vi "MQTT_PubAck_Read.vi"(8 "error in (no error)":errorcluster, 11 "SSL_Connection":T1) -> (0 "error out":errorcluster, 2 "Message ID":u16=10 format="%x", 3 "SSL_Connection":T1)   [LabVIEW 2018, in "AWS_IoT.lvlib"]
doc: "© 2015 - daq.io, LLC - Peter Adelhardt"
uses:
  AWS_IoT.lvlib
  Controls/SSL_Connection.ctl
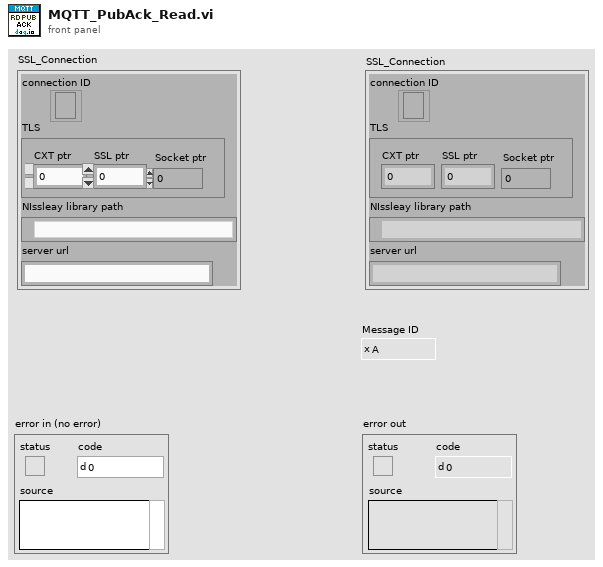
[diagram p1: front panel]
types:
  T1 = typedef "AWS_IoT.lvlib/SSL_Connection.ctl" = cluster{"connection ID":refnum<k5>, "TLS":cluster{"CXT ptr":i32, "SSL ptr":i32, "Socket ptr":i32}, "NIssleay library path":path, "server url":string}
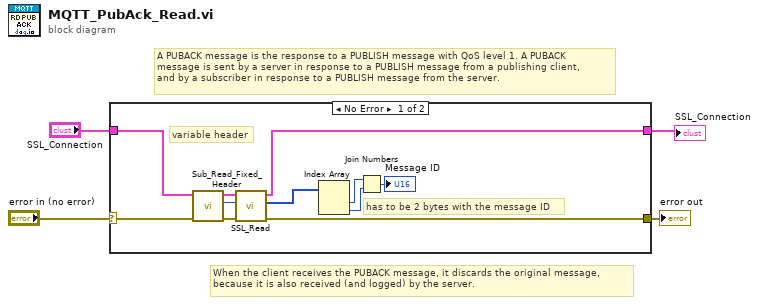
[diagram p0: block diagram]
diagram:
  # "When the client receives the PUBACK message, it discards the original message,\nbecause it is also received (and logged) by the server."
  # "A PUBACK message is the response to a PUBLISH message with QoS level 1. A PUBACK\nmessage is sent by a server in response to a PUBLISH message from a publishing client,\nand by a subscriber in response to a PUBLISH message from the server."
  n1 = case shown="No Error" "error in (no error)" {
    selector: "error in (no error)" -> [w15 w17]
    tunnel: [w8 w17] -> w3
    tunnel: "SSL_Connection" -> [w6 w16]
    tunnel: [w5 w16] -> w1
    frame No Error {
      # "has to be 2 bytes with the message ID"
      # "variable header"
      n2 = call "Sub_Read_Fixed_Header.vi"("error in (no error)"=w15, "SSL_Connection"=w6) -> ("error out"=w11:errorcluster, "Remaining Length"=w9:u32, "SSL_Connection"=w10:T1)  [unwired: 3 in, 4 out]
      n3 = call "SSL_Read.vi"("error in (no error)"=w11, "bytes to read"=w9, "SSL_Connection"=w10) -> ("error out"=w8:errorcluster, "data out"=w7:u8[], "SSL_Connection"=w5:T1)  [unwired: 5 in, 1 out]
      n4 = Index Array(array=w7) -> (element #1=w13:u8, element #2=w14:u8)  [unwired: 2 in]
      n5 = Join Numbers(hi=w13, lo=w14) -> ((hi.lo)=→"Message ID":u16)
    }
    frame Error {
    }
  }
  "error out" <- w3
  "SSL_Connection" <- w1
